vi "Get Output Mode.vi"(8 "error in (no error)":errorcluster, 11 "VISA resource name":refnum<visa-resource-name>) -> (0 "error out":errorcluster, 2 "Output Mode":i32, 3 "VISA resource name out":refnum<visa-resource-name>)   [LabVIEW 2013, in "Fluke 5XXX Series Multicalibrators.lvlib"]
doc: "This VI returns state of the Calibrator output. When On, the Calibrator is operating. When Off, it is in standbay."
uses:
  Fluke 5XXX Series Multicalibrators.lvlib
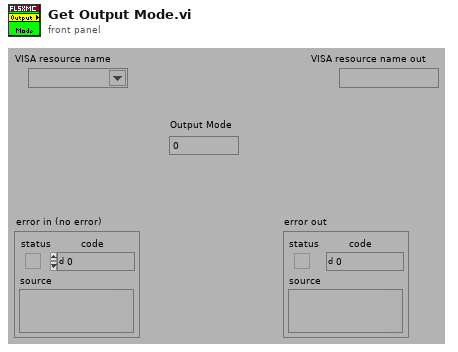
[diagram p1: front panel]
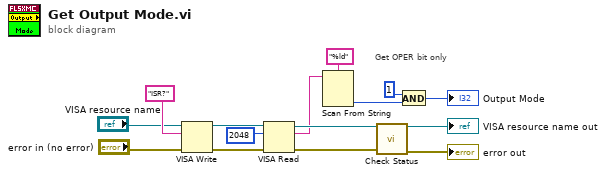
[diagram p0: block diagram]
diagram:
  # "Get OPER bit only"
  n1 = VISA Write(VISA resource name="VISA resource name", write buffer="ISR?", error in (no error)="error in (no error)") -> (VISA resource name out=w14:refnum<visa-resource-name>, error out=w13:errorcluster)  [unwired: 1 out]
  n2 = VISA Read(VISA resource name=w14, byte count=u32 2048 ("byte count (0)"), error in (no error)=w13) -> (VISA resource name out=w9:refnum<visa-resource-name>, read buffer=w8:string, error out=w10:errorcluster)  [unwired: 1 out]
  n3 = Scan From String(format string="%ld", input string=w8) -> (output 1=w2:i32)  [unwired: 3 in, 3 out]
  n4 = call "Check Status.vi"("VISA resource name"=w9, "error in (no error)"=w10) -> ("VISA resource name out"=→"VISA resource name out":refnum<visa-resource-name>, "error out"=→"error out":errorcluster)  [unwired: 12 in]
  n5 = And(x=1, y=w2) -> (x .and. y?=→"Output Mode":i32)
